vi "MP-ThicknessGauge.vi"() -> ()   [LabVIEW 2015]
uses:
  <instrlib>/MicroPulse/Public/Data/Datatypes/MP - data formatting.ctl
  <instrlib>/MicroPulse/Public/Data/Datatypes/MP - amplitude reporting mode.ctl
  <instrlib>/MicroPulse/Public/Data/Datatypes/MP - averaging.ctl
  <instrlib>/MicroPulse/Public/Data/Datatypes/MP - transmit parameters.ctl
  <instrlib>/MicroPulse/Public/Data/Datatypes/MP - pulser voltage.ctl
  <instrlib>/MicroPulse/Public/Data/Datatypes/MP - pulse damping.ctl
  <instrlib>/MicroPulse/Public/Data/Datatypes/MP - test parameters.ctl
  <instrlib>/MicroPulse/Public/Data/Datatypes/MP - receive parameters.ctl
  <instrlib>/MicroPulse/Public/Data/Datatypes/MP - display gate.ctl
  <instrlib>/MicroPulse/Public/Data/Datatypes/MP - waveform type.ctl
  <instrlib>/MicroPulse/Public/Data/Datatypes/MP - analogue filter.ctl
  <instrlib>/MicroPulse/Public/Data/Datatypes/MP - frequency filter.ctl
  <instrlib>/MicroPulse/Public/Data/Datatypes/MP - digital filtering.ctl
  <instrlib>/MicroPulse/Public/Data/Datatypes/MP - high pass filter.ctl
  <instrlib>/MicroPulse/Public/Data/Datatypes/MP - low pass filter.ctl
  <instrlib>/MicroPulse/Public/Data/Datatypes/TCP config.ctl
  <instrlib>/MicroPulse/Public/Data/Datatypes/MP - multi-gate inspection.ctl
  <instrlib>/MicroPulse/Public/Data/Datatypes/MP - multigate inspection gate parameters.ctl
  <instrlib>/MicroPulse/Public/Data/Datatypes/MP - hysteresis level.ctl
  <instrlib>/MicroPulse/Public/Data/Datatypes/MP - multigate mode.ctl
  <instrlib>/MicroPulse/Public/Data/Datatypes/MP - data output format.ctl
  <instrlib>/MicroPulse/Public/Data/Datatypes/MP - instrument type.ctl
  <instrlib>/MicroPulse/Public/Data/Datatypes/MP - sample frequency.ctl
  <instrlib>/MicroPulse/Public/Data/Datatypes/MP - echo gate mode.ctl
  <vilib>/Analysis/baseanly.llb/Mean (DBL).vi
  <instrlib>/MicroPulse/MicroPulse_Driver.lvlib
  <vilib>/Analysis/NI_AALBase.lvlib
panel:
  in  "Calculate":enum16{"Speed Of Sound", "Thickness"}(ring)
  out "Calc Tab":enum32{"Speed Of Sound", "Thickness"}(tab)
  in  "Sample thickness":dbl=12.0 format="%#_6f mm"
  out "SOS":dbl[](array[numeric]) format="%#.2f m/s"
  out "Average SOS":dbl format="%#.2f m/s"
  in  "Speed Of Sound":dbl=5790.0 format="%#_6f m/s"
  out "Thickness":dbl[](array[numeric]) format="%#.2f mm"
  out "Average Thickness":dbl format="%#.2f mm"
  in  "Tab Control":enum32{"Basics", "Test Parameters", "Gates"}(tab)
  in  "Test Parameters":T1={"Test No."=1, "Tx Channel"=1, "Rx Channel"=1} {"Rx Channel" min=1 max=1024; "Tx Channel" min=1 max=1024}
  in  "PRF":u16=50 caption="[PRF]" min=1 max=20000 step=100 format="%dHz"
  in  "Data Output Format":T2=enum."8-bit Mode" caption="[DOF]"
  in  "TCP config":T3={"Connection ID"=refnum, "IP address"="10.1.1.2", "host port"=1067, "OC timeout"=5000, "Read timeout"=2000, "Write timeout"=100} {"Write timeout" format="%dms"; "Read timeout" format="%dms"; "OC timeout" format="%dms"}
  in  "Data Formatting":T4={"Amplitude Mode"=enum."Peaks + Ascan for Multigate", "Averaging"=enum."None", "Coupling Level"=0} {"Coupling Level" max=4095 step=1}
  in  "Transmit Parameters":T7={"Pulse Voltage"=enum."50V", "Pulse Shape"={"Damping"=enum."660W", "Width"=100}} {"Pulse Shape"."Width" min=16 max=1010 step=50 format="%.0fns"}
  in  "Receive Parameters":T10={"Display Gate"={"Start"=0.0, "Length"=50.0}, "Delay"=0.0, "Waveform Type"=enum."Rectified Signal", "Gain"=7.5, "Analogue Filtering"={"Bandpass"=enum."5MHz Bandpass", "Smoothing"=7}, "Digital Filtering"={"High Pass Filter"=enum."None", "Low Pass Filter"=enum."None"}} {"Delay" format="%#_g us"; "Display Gate"."Length" min=0.0 max=64000.0 step=1.0 format="%#_g us"; "Display Gate"."Start" min=0.0 max=64000.0 step=1.0 format="%#_g us"; "Analogue Filtering"."Smoothing" min=1 max=11 step=1; "Gain" min=-6.0 max=70.0 step=0.25 format="%.2fdB"}
  in  "Multi Gate Inspection":T18={"Gate 1"={"Start (us)"=8.0, "Length (us)"=4.0, "Threshold"=40, "Enabled?"=TRUE, "Max # Peaks"=8, "Hysteresis"=enum."6dB", "Mode"=enum."Largest Peak In Gate", "Inverted?"=FALSE, "Colour "=16716306}, "Gate 2"={"Start (us)"=16.0, "Length (us)"=4.0, "Threshold"=40, "Enabled?"=TRUE, "Max # Peaks"=8, "Hysteresis"=enum."6dB", "Mode"=enum."Largest Peak In Gate", "Inverted?"=FALSE, "Colour "=641024}, "Gate 3"={"Start (us)"=24.0, "Length (us)"=4.0, "Threshold"=40, "Enabled?"=TRUE, "Max # Peaks"=8, "Hysteresis"=enum."6dB", "Mode"=enum."Largest Peak In Gate", "Inverted?"=FALSE, "Colour "=4532}, "Gate 4"={"Start (us)"=34.0, "Length (us)"=4.0, "Threshold"=40, "Enabled?"=TRUE, "Max # Peaks"=8, "Hysteresis"=enum."6dB", "Mode"=enum."Largest Peak In Gate", "Inverted?"=FALSE, "Colour "=8978537}} {"Gate 4"."Max # Peaks" min=1 max=80 step=1; "Gate 4"."Threshold" min=10 step=10; "Gate 4"."Length (us)" min=0.0 max=96000.0 step=1.0; "Gate 4"."Start (us)" min=0.0 max=64000.0 step=1.0; "Gate 3"."Max # Peaks" min=1 max=80 step=1; "Gate 3"."Threshold" min=10 step=10; "Gate 3"."Length (us)" min=0.0 max=96000.0 step=1.0; "Gate 3"."Start (us)" min=0.0 max=64000.0 step=1.0; "Gate 2"."Max # Peaks" min=1 max=80 step=1; "Gate 2"."Threshold" min=10 step=10; "Gate 2"."Length (us)" min=0.0 max=96000.0 step=1.0; "Gate 2"."Start (us)" min=0.0 max=64000.0 step=1.0; "Gate 1"."Max # Peaks" min=1 max=80 step=1; "Gate 1"."Threshold" min=10 step=10; "Gate 1"."Length (us)" min=0.0 max=96000.0 step=1.0; "Gate 1"."Start (us)" min=0.0 max=64000.0 step=1.0}
  out "Sample Frequency":T22=enum."100MHz"
  out "Instrument Type":T23=enum."Simulated Data"
  in  "Gate No.":i32=1 min=1 max=4
  out "peak data":cluster{"Time (us)":dbl[], "Level":u16[]}={"Time (us)"=[9.05], "Level"=[53]} {"Time (us)" format="%_6g"}
  out "A-Scan + Peaks":cluster{"timebase":dbl[], "data":u16[]}[](graph)=[{"timebase"=array[5000 elements], "data"=array[5000 elements]}, {"timebase"=[9.05], "data"=[53]}, {"timebase"=[17.71], "data"=[65]}, {"timebase"=[26.28], "data"=[48]}, {"timebase"=[34.87], "data"=[49]}]
  in  "Single Scan":bool
  in  "Stop Acquisition":bool
  in  "Start Acquisition":bool
  out "Command List":string="ENCM 2\r\nDOF 1\r\nPRF 50\r\nNUM 1\r\nTXN 1 1\r\nRXN 1 1\r\nAMP 1 32 \r\nPSV 1 50\r\nPDW 1 0 250\r\nGAT 1 0 5000\r\nDLY 1 0\r\nAWF 1 0\r\nGAN 1 137\r\nFRD 1 0 0\r\nETM 1 0\r\nGMT 1 1 800 1200\r\nHMS 1 1 2\r\nAMM 1 1 10\r\nPMG 1 1 8\r\nGIN 1 1 0\r\nUML 1 1 40\r\nAG.GMT_COL 1 1 FF1212\r\nGMT 1 2 1600 2000\r\nHMS 1 2 2\r\nAMM 1 2 10\r\nPMG 1 2 8\r\nGIN 1 2 0\r\nUML 1 2 40\r\nAG.GMT_COL 1 2 09C800\r\nGMT 1 3 2400 2800\r\nHMS 1 3 2\r\nAMM 1 3 10\r\nPMG 1 3 8\r\nGIN 1 3 0\r\nUML 1 3 40\r\nAG.GMT_COL 1 3 0011B4\r\nGMT 1 4 3400 3800\r\nHMS 1 4 2\r\nAMM 1 4 10\r\nPMG 1 4 8\r\nGIN 1 4 0\r\nUML 1 4 40\r\nAG.GMT_COL 1 4 890069\r"
  in  "QUIT":bool
  out "running average PRF":dbl=49.99631559070177 format="%0.2f"
  out "live error out":errorcluster={"status"=FALSE, "code"=56, "source"="TCP read timeout"}
  out "message count":i32=1
  out "System Messages":string="11:55:31\n------------------\nSTX 1 Completed\n------------------\nBuffer Cleared Successfully\n\n"
  # "MP Thickness Gauge\n\nSet all controls to the required values\nbefore running the VI.\n\nWhile running, test parameters may be changed."
  # "Place gates on the first four echos."
  # "Channels MUST be set BEFORE running"
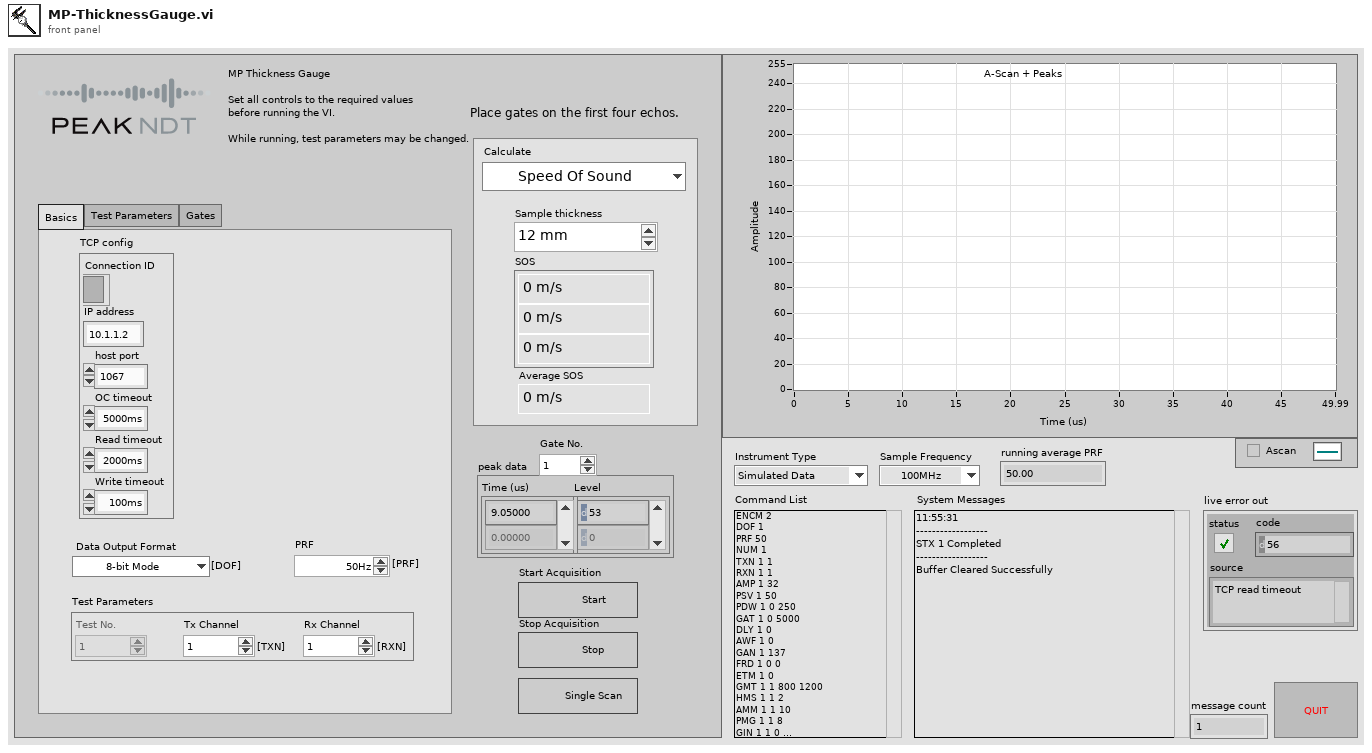
[diagram p1: front panel]
types:
  T1 = typedef "MicroPulse_Driver.lvlib/MP - test parameters.ctl" = cluster{"Test No.":u32, "Tx Channel":u32, "Rx Channel":u32}
  T2 = typedef "MicroPulse_Driver.lvlib/MP - data output format.ctl" = enum16{"", "8-bit Mode", "10-bit Mode", "12-bit Mode", "16-bit Mode", "8-bit Log Mode", "12-bit Packed Mode"}
  T3 = typedef "MicroPulse_Driver.lvlib/TCP config.ctl" = cluster{"Connection ID":refnum<k5>, "IP address":string, "host port":u16, "OC timeout":i32, "Read timeout":i32, "Write timeout":i32}
  T4 = typedef "MicroPulse_Driver.lvlib/MP - data formatting.ctl" = cluster{"Amplitude Mode":T5, "Averaging":T6, "Coupling Level":u32}
  T5 = typedef "MicroPulse_Driver.lvlib/MP - amplitude reporting mode.ctl" = enum16{"1st Peak in gate", "Maximum Peak in gate", "All Peaks", "Ascan Data", "1st Threshold Crossing Peak", "Ascan + Peaks", "All Peaks for Multigate", "Peaks + Ascan for Multigate", "Peaks + P_Ascan for Multigate", "Full Matrix Capture"}
  T6 = typedef "MicroPulse_Driver.lvlib/MP - averaging.ctl" = enum16{"None", "2", "4", "8", "16", "32", "64", "128", "256"}
  T7 = typedef "MicroPulse_Driver.lvlib/MP - transmit parameters.ctl" = cluster{"Pulse Voltage":T8, "Pulse Shape":cluster{"Damping":T9, "Width":u32}}
  T8 = typedef "MicroPulse_Driver.lvlib/MP - pulser voltage.ctl" = enum16{"50V", "100V", "150V", "200V", "250V", "300V"}
  T9 = typedef "MicroPulse_Driver.lvlib/MP - pulse damping.ctl" = enum16{"660W", "458W", "220W", "149W", "102W", "82W", "63W", "51W"}
  T10 = typedef "MicroPulse_Driver.lvlib/MP - receive parameters.ctl" = cluster{"Display Gate":T11, "Delay":dbl, "Waveform Type":T12, "Gain":dbl, "Analogue Filtering":T13, "Digital Filtering":T15}
  T11 = typedef "MicroPulse_Driver.lvlib/MP - display gate.ctl" = cluster{"Start":dbl, "Length":dbl}
  T12 = typedef "MicroPulse_Driver.lvlib/MP - waveform type.ctl" = enum16{"Rectified Signal", "RF Signal", "+Half Wave", "-Half Wave"}
  T13 = typedef "MicroPulse_Driver.lvlib/MP - analogue filter.ctl" = cluster{"Bandpass":T14, "Smoothing":u16}
  T14 = typedef "MicroPulse_Driver.lvlib/MP - frequency filter.ctl" = enum16{"No change", "1MHz Bandpass", "2MHz Bandpass", "4MHz Bandpass", "5MHz Bandpass", "10MHz Bandpass", "2.5-18MHz Broadband", "0.75-12MHz  Broadband", "0.5MHz Bandpass", "5MHz 2nd Order TOFD", "10MHz 2nd Order TOFD", "3.0-25MHz Broadband", "3.0-30MHz Broadband"}
  T15 = typedef "MicroPulse_Driver.lvlib/MP - digital filtering.ctl" = cluster{"High Pass Filter":T16, "Low Pass Filter":T17}
  T16 = typedef "MicroPulse_Driver.lvlib/MP - high pass filter.ctl" = enum16{"None", "0.7MHz", "1.5MHz", "4.0MHz", "7.5MHz", "10.0MHz", "User Defined"}
  T17 = typedef "MicroPulse_Driver.lvlib/MP - low pass filter.ctl" = enum16{"None", "1.8MHz", "3.0MHz", "6.0MHz", "8.0MHz", "12.0MHz", "User Defined"}
  T18 = typedef "MicroPulse_Driver.lvlib/MP - multi-gate inspection.ctl" = cluster{"Gate 1":T19, "Gate 2":T19, "Gate 3":T19, "Gate 4":T19}
  T19 = typedef "MicroPulse_Driver.lvlib/MP - multigate inspection gate parameters.ctl" = cluster{"Start (us)":dbl, "Length (us)":dbl, "Threshold":u16, "Enabled?":bool, "Max # Peaks":u16, "Hysteresis":T20, "Mode":T21, "Inverted?":bool, "Colour ":u32}
  T20 = typedef "MicroPulse_Driver.lvlib/MP - hysteresis level.ctl" = enum16{"None", "3dB", "6dB", "9dB", "12dB"}
  T21 = typedef "MicroPulse_Driver.lvlib/MP - multigate mode.ctl" = enum16{"1st Peak in Gate", "Largest Peak In Gate", "All Peaks In Gate", "1st Threshold Crossing"}
  T22 = typedef "MicroPulse_Driver.lvlib/MP - sample frequency.ctl" = enum16{"Use Default", "200MHz (LT2 only)", "100MHz", "50MHz", "25MHz", "10MHz"}
  T23 = typedef "MicroPulse_Driver.lvlib/MP - instrument type.ctl" = enum16{"MicroPulse 5", "LT1", "LT2", "LTPA", "MPLT", "MicroPulse 6", "PipeScanner", "<MicroPulse>", "Micropulse 4", "Simulated Data"}
  T24 = typedef "MicroPulse_Driver.lvlib/MP - echo gate mode.ctl" = enum16{"Echo Trigger OFF", "Echo Gate Display Mode", "Echo Trigger ON", "Multi Gate or FMC Mode", "Reserved", "PA - Echo Trigger ON"}
  T25 = typedef "MicroPulse_Driver.lvlib/MP-Registry Data-Cluster.ctl" = cluster{"Instrument Type":T23, "Serial #":u64, "Sample Frequency":T22, "dt (us)":dbl, "DOF":T2, "Material Velocity":dbl, "Asynch Reads":T26, "NUM of Tests":u32, "System Details":T27, "Gates":T29[], "Encoders":T31[], "CMD LUT":variant, "Command List":string}
  T26 = typedef "MicroPulse_Driver.lvlib/MP - asynch read mode.ctl" = enum16{"Disabled", "Enabled"}
  T27 = typedef "MicroPulse_Driver.lvlib/MP - general system status.ctl" = cluster{"System Type":T23, "Serial No.":u64, "Channels":cluster{"Conv":u8, "PA":u16, "Extra":u32}, "Sample Frequency":cluster{"Default":u8, "Actual":u8}, "Software Versions":string, "Data Output Format":cluster{"Default":T2, "Actual":T2}, "Temperatures":cluster{"System":u8, "Processor":u8, "Slave Sys":u8, "Slave Proc":u8}, "Tx Buffer Size":u32, "System Error":string, "No. of Cards":u8, "DAC Gain":i16, "Uptimes":cluster{"since Power":u32, "since RSTS":u32, "since SRST":u32}, "Voltages":cluster{"Nominal":dbl, "Measured":dbl, "Difference":dbl}[], "Interface Cards":T28[]}
  T28 = typedef "MicroPulse_Driver.lvlib/MP - interface card status.ctl" = cluster{"Status":u8, "Map":u8, "Board - T":u8, "FPGA - T":u8, "PAIF Status":string, "Version":string}
  T29 = typedef "MicroPulse_Driver.lvlib/MP - Registry Gates.ctl" = cluster{"Display Gate":T11, "ETM Mode":T24, "Echo Gate":T30, "Insp Gates":T19[]}
  T30 = typedef "MicroPulse_Driver.lvlib/MP - echo gate parameters.ctl" = cluster{"Start (us)":dbl, "Length (us)":dbl, "Threshold":u16, "Colour":u32}
  T31 = typedef "MicroPulse_Driver.lvlib/MP - encoder settings.ctl" = cluster{"Encoder Type":T32, "Counts/mm":u32, "Enable Termination?":bool, "Multiplier":u32, "Backlash Period (s)":dbl, "Encoder Filter":u32}
  T32 = typedef "MicroPulse_Driver.lvlib/MP - encoder type.ctl" = enum16{"Quadrature", "Step/Direction"}
  T33 = typedef "MicroPulse_Driver.lvlib/MP - scan data info.ctl" = cluster{"Message Header":u16, "Error Message":u16, "Test No.":u32, "Channel No.":u8, "Sweep No.":u32, "Gate No.":u32, "DOF":T2, "retain data":T34, "scan data":u16[], "scan length":i32, "scan index":i32, "peak data":cluster{"timebase":u16[], "data":u16[]}, "#peaks":i32, "PRF":dbl, "IP":cluster{"Axis No.":u8, "Location":u32, "MIP location":u32, "MIP?":bool}, "echo range":u16, "ETG":bool, "CAL 0 complete":bool, "Axis Positions":T35}
  T34 = typedef "MicroPulse_Driver.lvlib/MP - retain scan.ctl" = enum16{"None", "Ascan", "Peaks"}
  T35 = typedef "MicroPulse_Driver.lvlib/MP - axis positions (LLC).ctl" = cluster{"Axis 1":u32, "Axis 2":u32, "Axis 3":u32, "Axis 4":u32, "Status":u8}
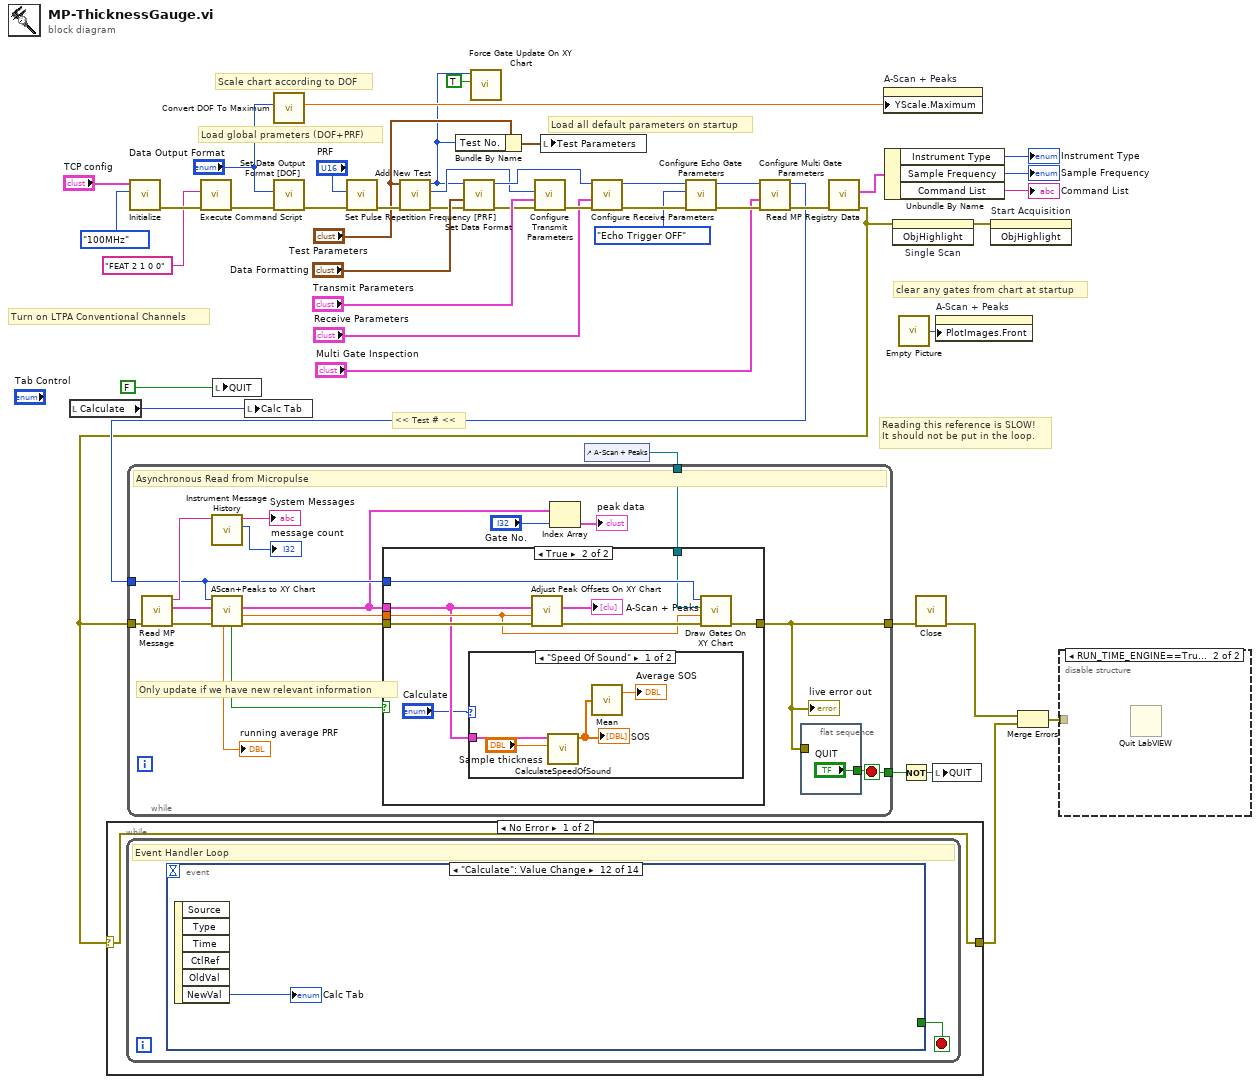
[diagram p0: block diagram]
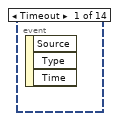
[diagram p3: hidden frame]
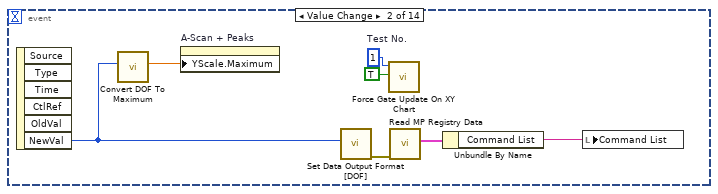
[diagram p4: hidden frame]
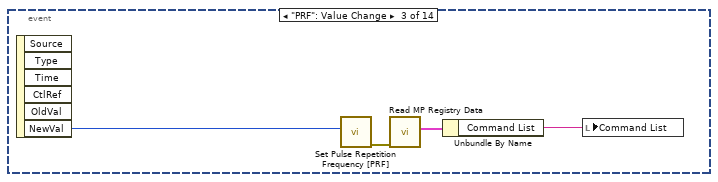
[diagram p5: hidden frame]
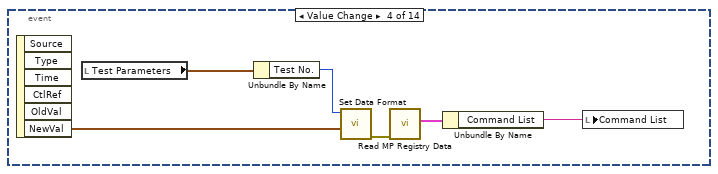
[diagram p6: hidden frame]
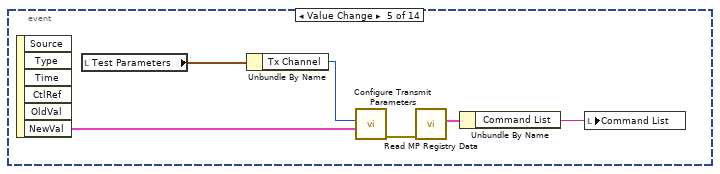
[diagram p7: hidden frame]
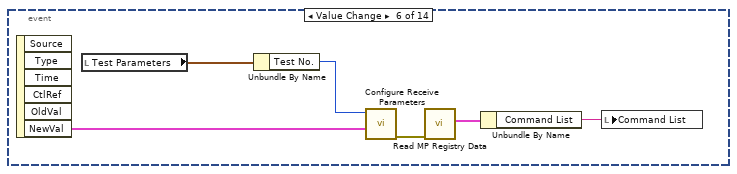
[diagram p8: hidden frame]
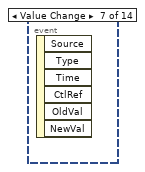
[diagram p9: hidden frame]
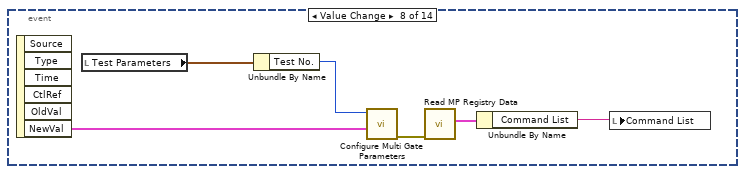
[diagram p10: hidden frame]
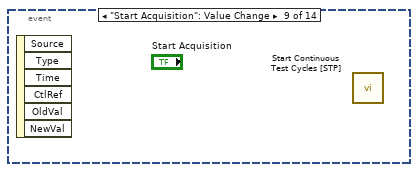
[diagram p11: hidden frame]
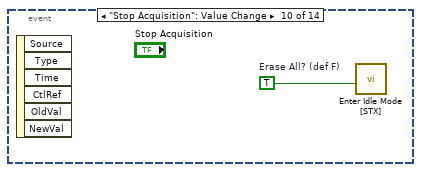
[diagram p12: hidden frame]
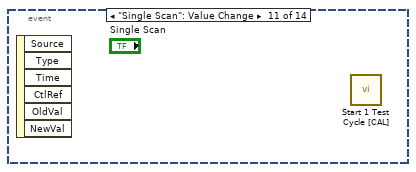
[diagram p13: hidden frame]
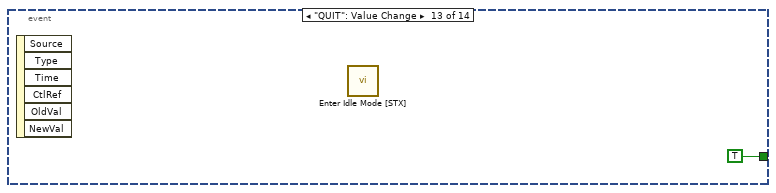
[diagram p14: hidden frame]
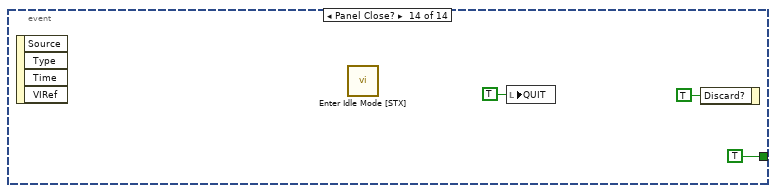
[diagram p15: hidden frame]
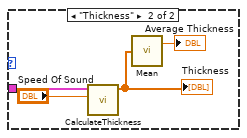
[diagram p18: hidden frame]
diagram:
  # "Turn on LTPA Conventional Channels"
  # "Scale chart according to DOF"
  # "Load global prameters (DOF+PRF)"
  # "Reading this reference is SLOW!\nIt should not be put in the loop."
  # "clear any gates from chart at startup"
  # "<< Test # <<"
  # "Load all default parameters on startup"
  n1 = local read "Calculate"() -> (w5:enum16{"Speed Of Sound", "Thickness"})
  n2 = call <instrlib>:"Initialize.vi"("Sample Frequency"=MP_-_sample_frequency."100MHz", "TCP config"="TCP config") -> ("error out"=w25:errorcluster)  [unwired: 8 in, 1 out]
  n3 = call <instrlib>:"Execute Command Script.vi"("error in (no error)"=w25, "String in"="FEAT 2 1 0 0") -> ("error out"=w2:errorcluster)  [unwired: 7 in, 2 out]
  n4 = local write "QUIT"(FALSE ("QUIT")) -> ()
  n5 = local write "Calc Tab"(w5) -> ()
  n6 = call <instrlib>:"Convert DOF To Maximum.vi"("Data Output Format"="Data Output Format") -> ("Data Maximum"=w15:dbl)  [unwired: 10 in]
  n7 = call <instrlib>:"Set Data Output Format [DOF].vi"("error in (no error)"=w2, "Mode"="Data Output Format") -> ("error out"=w24:errorcluster)  [unwired: 8 in, 1 out]
  n8 = call <instrlib>:"Set Pulse Repetition Frequency [PRF].vi"("error in (no error)"=w24, "Frequency (Hz)"="PRF") -> ("error out"=w23:errorcluster)  [unwired: 8 in, 1 out]
  n9 = call <instrlib>:"Add New Test.vi"("error in (no error)"=w23, "Test Parameters"="Test Parameters") -> ("error out"=w33:errorcluster, "Tx Channel out"=w20:u32, "Test No. out"=w14:u32)  [unwired: 6 in, 1 out]
  n10 = Bundle By Name(cluster="Test Parameters", "Test No."=w14) -> (w19:T1)
  n11 = call <instrlib>:"Set Data Format.vi"("error in (no error)"=w33, "Data Formatting"="Data Formatting", "Test No."=w14) -> ("error out"=w42:errorcluster, "Test No. out"=w35:u32)  [unwired: 6 in, 1 out]
  n12 = call <instrlib>:"Force Gate Update On XY Chart.vi"("Set?"=TRUE, "Test No."=w14) -> ()  [unwired: 7 in, 3 out]
  n13 = call <instrlib>:"Configure Transmit Parameters.vi"("error in (no error)"=w42, "Transmit Parameters"="Transmit Parameters", "Tx Channel"=w20) -> ("error out"=w43:errorcluster)  [unwired: 7 in, 1 out]
  n14 = local write "Test Parameters"(w19) -> ()
  n15 = control-ref of="A-Scan + Peaks"() -> (w26:refnum<vi>)
  n16 = call <instrlib>:"Configure Receive Parameters.vi"("error in (no error)"=w43, "Receive Parameters"="Receive Parameters", "Test No."=w35) -> ("error out"=w41:errorcluster, "Test No. out"=w36:u32)  [unwired: 6 in, 1 out]
  n17 = call <instrlib>:"Configure Echo Gate Parameters.vi"("error in (no error)"=w41, "Echo Trigger Mode"=MP_-_echo_gate_mode."Echo Trigger OFF", "Test Number"=w36) -> ("error out"=w39:errorcluster, "Test Number Out"=w34:u32)  [unwired: 6 in, 1 out]
  n18 = call <instrlib>:"Configure Multi Gate Parameters.vi"("error in (no error)"=w39, "Multi Gate Inspection"="Multi Gate Inspection", "Test Number"=w34) -> ("error out"=w38:errorcluster, "Test Number out"=w32:u32)  [unwired: 6 in, 1 out]
  n19 = call <instrlib>:"Read MP Registry Data.vi"("error in (no error)"=w38) -> ("error out"=w28:errorcluster, "Micropulse Data"=w30:T25)  [unwired: 7 in, 2 out]
  n20 = case shown="No Error" w28 {
    selector: w28 -> [w47 w90]
    tunnel: [w47 w90] -> w7
    frame No Error {
      n21 = while {
        stop <- w48 stop-if-true
        # "Event Handler Loop"
        n22 = event shown="[11] \"Calculate\": Value Change" {
          selector: _ -> [_ _ _ _ _ _ _ _ _ _ _ _ _ _]
          dyn-events: _ -> [_ _ _ _ _ _ _ _ _ _ _ _ _ _]
          timeout: _ -> [_ _ _ _ _ _ _ _ _ _ _ _ _ _]
          tunnel: [_ _ _ _ _ _ _ _ _ _ _ _ TRUE ("stop") TRUE ("stop")] -> w48
          event Timeout {
            n23 = event-data() -> ()  [unwired: 1 in, 3 out]
          }
          event Value Change {
            w50 = u32 1  # Test No.
            n24 = event-data() -> ("NewVal"=w51:T2)  [unwired: 1 in, 5 out]
            n25 = call <instrlib>:"Convert DOF To Maximum.vi"("Data Output Format"=w51) -> ("Data Maximum"=w52:dbl)  [unwired: 10 in]
            n26 = property on="A-Scan + Peaks" class="XYGraph (strict)"("YScale.Maximum"=w52) -> ()  [unwired: 2 in, 2 out]
            n27 = call <instrlib>:"Set Data Output Format [DOF].vi"("Mode"=w51) -> ("error out"=w55:errorcluster)  [unwired: 9 in, 1 out]
            n28 = call <instrlib>:"Force Gate Update On XY Chart.vi"("Set?"=TRUE, "Test No."=w50) -> ()  [unwired: 7 in, 3 out]
            n29 = call <instrlib>:"Read MP Registry Data.vi"("error in (no error)"=w55) -> ("Micropulse Data"=w54:T25)  [unwired: 7 in, 3 out]
            n30 = Unbundle By Name(w54) -> ("Command List"=w53:string)
            n31 = local write "Command List"(w53) -> ()
          }
          event "PRF": Value Change {
            n32 = event-data() -> ("NewVal"=w56:u16)  [unwired: 1 in, 5 out]
            n33 = call <instrlib>:"Set Pulse Repetition Frequency [PRF].vi"("Frequency (Hz)"=w56) -> ("error out"=w59:errorcluster)  [unwired: 9 in, 1 out]
            n34 = call <instrlib>:"Read MP Registry Data.vi"("error in (no error)"=w59) -> ("Micropulse Data"=w58:T25)  [unwired: 7 in, 3 out]
            n35 = Unbundle By Name(w58) -> ("Command List"=w57:string)
            n36 = local write "Command List"(w57) -> ()
          }
          event Value Change {
            n37 = event-data() -> ("NewVal"=w65:T4)  [unwired: 1 in, 5 out]
            n38 = local read "Test Parameters"() -> (w61:T1)
            n39 = Unbundle By Name(w61) -> ("Test No."=w60:u32)
            n40 = call <instrlib>:"Set Data Format.vi"("Data Formatting"=w65, "Test No."=w60) -> ("error out"=w64:errorcluster)  [unwired: 7 in, 2 out]
            n41 = call <instrlib>:"Read MP Registry Data.vi"("error in (no error)"=w64) -> ("Micropulse Data"=w63:T25)  [unwired: 7 in, 3 out]
            n42 = Unbundle By Name(w63) -> ("Command List"=w62:string)
            n43 = local write "Command List"(w62) -> ()
          }
          event Value Change {
            n44 = event-data() -> ("NewVal"=w70:T7)  [unwired: 1 in, 5 out]
            n45 = local read "Test Parameters"() -> (w71:T1)
            n46 = Unbundle By Name(w71) -> ("Tx Channel"=w69:u32)
            n47 = call <instrlib>:"Configure Transmit Parameters.vi"("Transmit Parameters"=w70, "Tx Channel"=w69) -> ("error out"=w67:errorcluster)  [unwired: 8 in, 1 out]
            n48 = call <instrlib>:"Read MP Registry Data.vi"("error in (no error)"=w67) -> ("Micropulse Data"=w68:T25)  [unwired: 7 in, 3 out]
            n49 = Unbundle By Name(w68) -> ("Command List"=w66:string)
            n50 = local write "Command List"(w66) -> ()
          }
          event Value Change {
            n51 = event-data() -> ("NewVal"=w75:T10)  [unwired: 1 in, 5 out]
            n52 = local read "Test Parameters"() -> (w77:T1)
            n53 = Unbundle By Name(w77) -> ("Test No."=w76:u32)
            n54 = call <instrlib>:"Configure Receive Parameters.vi"("Receive Parameters"=w75, "Test No."=w76) -> ("error out"=w74:errorcluster)  [unwired: 7 in, 2 out]
            n55 = call <instrlib>:"Read MP Registry Data.vi"("error in (no error)"=w74) -> ("Micropulse Data"=w72:T25)  [unwired: 7 in, 3 out]
            n56 = Unbundle By Name(w72) -> ("Command List"=w73:string)
            n57 = local write "Command List"(w73) -> ()
          }
          event Value Change {
            n58 = event-data() -> ()  [unwired: 1 in, 6 out]
          }
          event Value Change {
            n59 = event-data() -> ("NewVal"=w81:T18)  [unwired: 1 in, 5 out]
            n60 = local read "Test Parameters"() -> (w83:T1)
            n61 = Unbundle By Name(w83) -> ("Test No."=w82:u32)
            n62 = call <instrlib>:"Configure Multi Gate Parameters.vi"("Multi Gate Inspection"=w81, "Test Number"=w82) -> ("error out"=w80:errorcluster)  [unwired: 7 in, 2 out]
            n63 = call <instrlib>:"Read MP Registry Data.vi"("error in (no error)"=w80) -> ("Micropulse Data"=w79:T25)  [unwired: 7 in, 3 out]
            n64 = Unbundle By Name(w79) -> ("Command List"=w78:string)
            n65 = local write "Command List"(w78) -> ()
          }
          event "Start Acquisition": Value Change {
            n66 = event-data() -> ()  [unwired: 1 in, 6 out]
            n67 = call <instrlib>:"Start Continuous Test Cycles [STP].vi"() -> ()  [unwired: 10 in, 2 out]
          }
          event "Stop Acquisition": Value Change {
            w84 = TRUE  # Erase All? (def F)
            n68 = event-data() -> ()  [unwired: 1 in, 6 out]
            n69 = call <instrlib>:"Enter Idle Mode [STX].vi"("Erase All? (def T)"=w84) -> ()  [unwired: 9 in, 2 out]
          }
          event "Single Scan": Value Change {
            n70 = event-data() -> ()  [unwired: 1 in, 6 out]
            n71 = call <instrlib>:"Start 1 Test Cycle [CAL].vi"() -> ()  [unwired: 10 in, 2 out]
          }
          event "Calculate": Value Change {
            n72 = event-data() -> ("NewVal"=→"Calc Tab":enum16{"Speed Of Sound", "Thickness"})  [unwired: 1 in, 5 out]
          }
          event "QUIT": Value Change {
            n73 = event-data() -> ()  [unwired: 1 in, 6 out]
            n74 = call <instrlib>:"Enter Idle Mode [STX].vi"() -> ()  [unwired: 10 in, 2 out]
          }
          event Panel Close? {
            n75 = event-data() -> ()  [unwired: 1 in, 4 out]
            n76 = call <instrlib>:"Enter Idle Mode [STX].vi"() -> ()  [unwired: 10 in, 2 out]
            n77 = local write "QUIT"(TRUE ("QUIT")) -> ()
            n78 = event-data("Discard?"=TRUE) -> ()  [unwired: 1 in, 1 out]
          }
        }
      }
    }
    frame Error {
    }
  }
  n79 = while {
    tunnel: w28 -> [w103]
    tunnel: w32 -> [w100]
    tunnel: w26 -> [w99]
    tunnel: [w92] -> w11
    tunnel: [w91] -> w4
    stop <- w91 stop-if-true
    # "Only update if we have new relevant information"
    # "Asynchronous Read from Micropulse"
    n80 = call <instrlib>:"Read MP Message.vi"("error in (no error)"=w103) -> ("error out"=w104:errorcluster, "scan data info"=w102:T33, "Instrument Message"=w106:string)  [unwired: 6 in, 2 out]
    n81 = call <instrlib>:"Instrument Message History.vi"("Instrument Message"=w106) -> ("Message Count"=→"message count":i32, "Message History out"=→"System Messages":string)  [unwired: 9 in]
    n82 = call <instrlib>:"AScan+Peaks to XY Chart.vi"("error in (no error)"=w104, "scan data info"=w102, "Test No."=w100) -> ("error out"=w101:errorcluster, "Echo Range (us)"=w98:dbl, "AScan+Peaks"=w93:cluster{"timebase":dbl[], "data":u16[]}[], "Update Indicators?"=w96:bool, "Running Average PRF"=→"running average PRF":dbl)  [unwired: 3 in, 1 out]
    n83 = case shown="True" w96 {
      tunnel: w101 -> [w108 w117]
      tunnel: [w108 w116] -> w92
      tunnel: w93 -> [_ w110]
      tunnel: w100 -> [_ w114]
      tunnel: w99 -> [_ w113]
      tunnel: w98 -> [_ w112]
      frame False {
      }
      frame True {
        n84 = case shown="\"Speed Of Sound\"" "Calculate" {
          tunnel: w110 -> [w120 w125]
          frame "Speed Of Sound" {
            n85 = call <instrlib>:"CalculateSpeedOfSound.vi"("Sample thickness"="Sample thickness", "AScan+Peaks"=w120) -> ("SOS"=w118:dbl[])  [unwired: 9 in]
            "SOS" <- w118
            n86 = call-poly <vilib>:"Mean.vi"("X"=w118) -> ("mean"=→"Average SOS":dbl)  [unwired: 1 out]
          }
          frame "Thickness" {
            n87 = call <instrlib>:"CalculateThickness.vi"("Speed Of Sound"="Speed Of Sound", "AScan+Peaks"=w125) -> ("Thickness [mm]"=w123:dbl[])  [unwired: 9 in]
            "Thickness" <- w123
            n88 = call-poly <vilib>:"Mean.vi"("X"=w123) -> ("mean"=→"Average Thickness":dbl)  [unwired: 1 out]
          }
        }
        n89 = call <instrlib>:"Adjust Peak Offsets On XY Chart.vi"("error in (no error)"=w117, "Echo Range in"=w112, "AScan+Peaks in"=w110) -> ("error out"=w115:errorcluster, "AScan+Peaks out"=→"A-Scan + Peaks":cluster{"timebase":dbl[], "data":u16[]}[])  [unwired: 7 in]
        n90 = call <instrlib>:"Draw Gates On XY Chart.vi"("error in (no error)"=w115, "Echo Range"=w112, "XYGraph in"=w113, "Test No."=w114) -> ("error out"=w116:errorcluster)  [unwired: 7 in]
      }
    }
    "live error out" <- w92
    n91 = Index Array(array=w93, index="Gate No.") -> (element=→"peak data":cluster{"timebase":dbl[], "data":u16[]})
    n92 = flat-sequence {
      tunnel: ["QUIT"] -> w91
      tunnel: w92 -> [_]
      frame #0 {
      }
    }
  }
  n93 = property on="A-Scan + Peaks" class="XYGraph (strict)"("YScale.Maximum"=w15) -> ()  [unwired: 2 in, 2 out]
  n94 = Unbundle By Name(w30) -> ("Instrument Type"=→"Instrument Type":T23, "Sample Frequency"=→"Sample Frequency":T22, "Command List"=→"Command List":string)
  n95 = invoke on="Single Scan" class="Bool" method="ObjHighlight"(error in=w28) -> (error out=w27:errorcluster)  [unwired: 2 in, 2 out]
  n96 = call "Empty Picture"() -> ("empty picture"=w37:picture)
  n97 = Not(x=w4) -> (.not. x?=w3:bool)
  n98 = call <instrlib>:"Close.vi"("error in (no error)"=w11) -> ("error out"=w8:errorcluster)  [unwired: 9 in, 1 out]
  n99 = local write "QUIT"(w3) -> ()
  n100 = property on="A-Scan + Peaks" class="XYGraph (strict)"("PlotImages.Front"=w37) -> ()  [unwired: 2 in, 2 out]
  n101 = invoke on="Start Acquisition" class="Bool" method="ObjHighlight"(error in=w27) -> ()  [unwired: 2 in, 3 out]
  n102 = Merge Errors(w8, w7) -> (w6:errorcluster)
  n103 = disable-structure shown="RUN_TIME_ENGINE==True" {
    disable-tunnel: w6 -> [_ _]
    frame condition #0 (active) {
    }
    frame condition #1 {
      n104 = Quit LabVIEW() -> ()  [unwired: 1 in]
    }
  }
